vi "MGCC_FntStaMach_Error_State_handle.vi"() -> ()   [LabVIEW 2016]
uses:
  Error Handler Command Input.ctl
  Abnormal Fault State Control (He Yin)/Sub_VIs/Fault_Abnormal_state.vi
panel:
  in  "Boolean 2":bool
  out "Boolean":bool
  in  "Session in":refnum<k21>
  out "result":bool
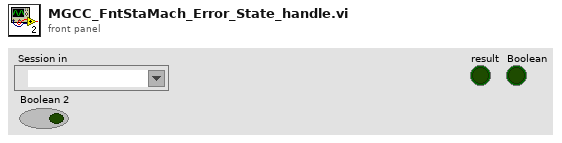
[diagram p1: front panel]
types:
  T1 = typedef "Error Handler Command Input.ctl" = enum16{"Initialize", "Handle Errors", "Report Errors"}
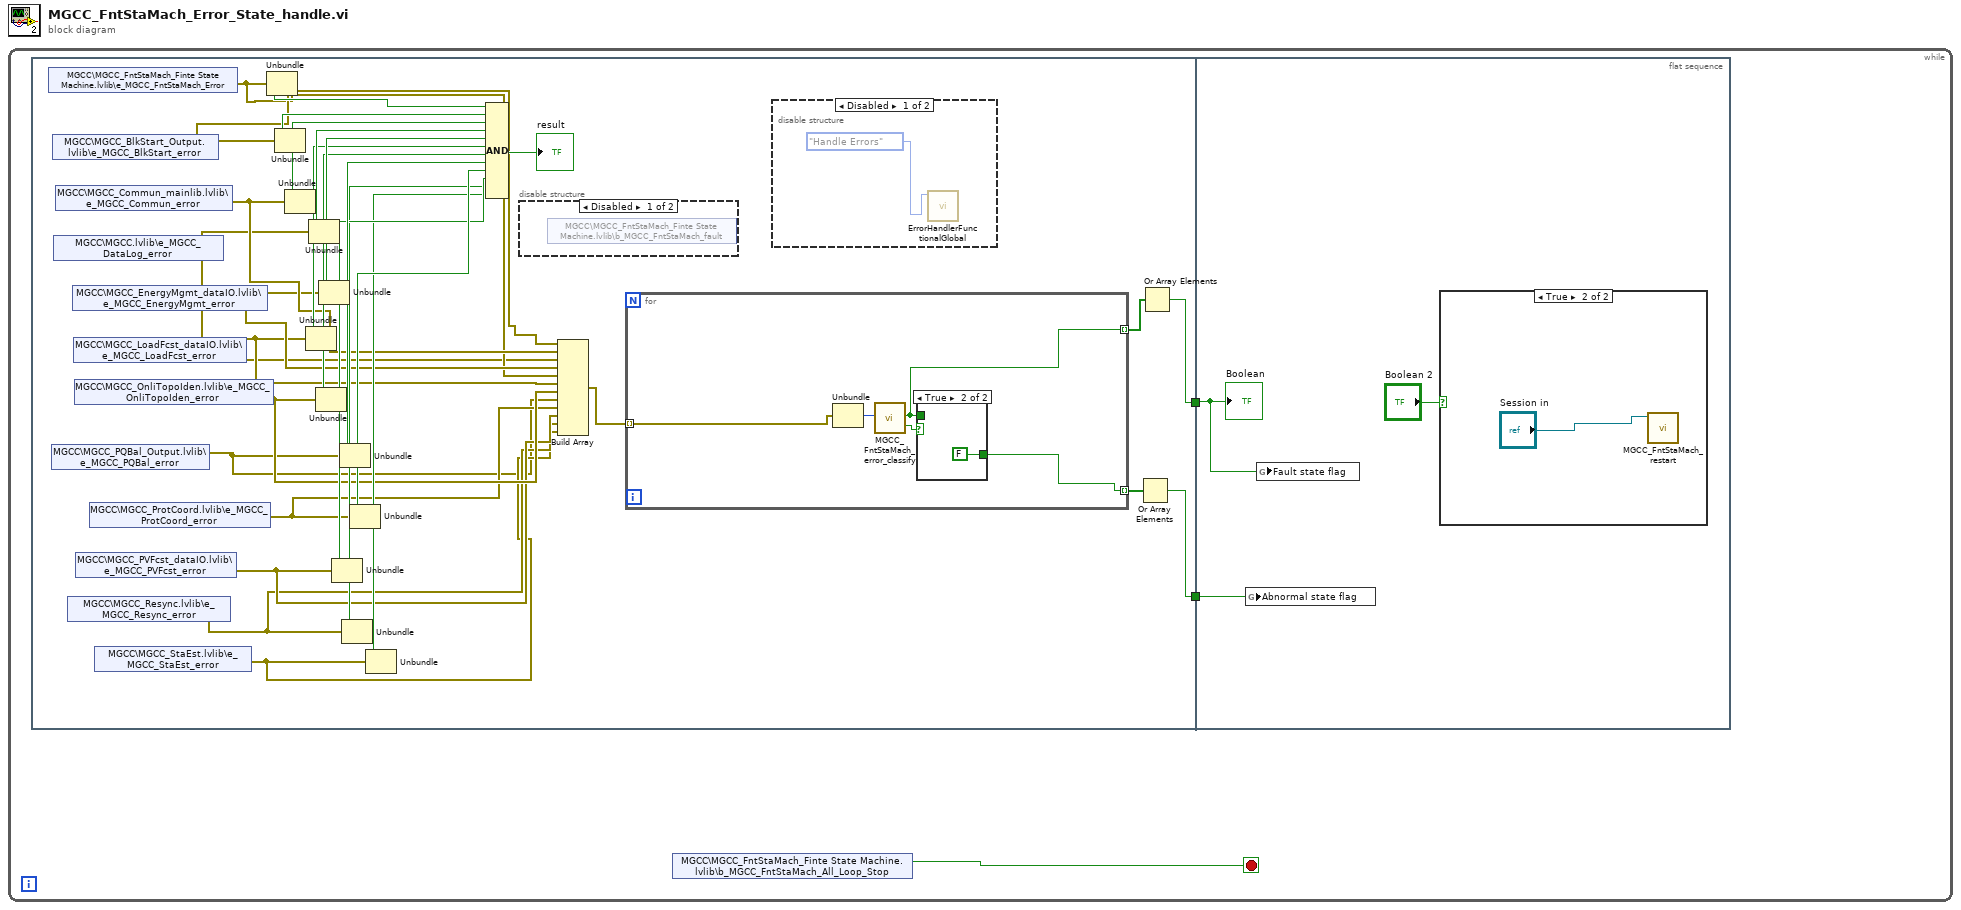
[diagram p0: block diagram]
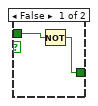
[diagram p3: hidden frame]
diagram:
  n1 = while {
    stop <- w3 stop-if-true
    n2 = flat-sequence {
      tunnel: [w5] -> w2
      tunnel: [w6] -> w1
      tunnel: w2 -> [w44]
      tunnel: w1 -> [w43]
      frame #0 {
        n3 = shared-variable "MGCC\\MGCC_FntStaMach_Finte State Machine.lvlib\\e_MGCC_FntStaMach_Error"() -> (w17:errorcluster)  [unwired: 1 in, 1 out]
        n4 = shared-variable "MGCC\\MGCC_PQBal_Output.lvlib\\e_MGCC_PQBal_error"() -> (w4:errorcluster)  [unwired: 1 in, 1 out]
        n5 = shared-variable "MGCC\\MGCC_BlkStart_Output.lvlib\\e_MGCC_BlkStart_error"() -> (w20:errorcluster)  [unwired: 1 in, 1 out]
        n6 = shared-variable "MGCC\\MGCC.lvlib\\e_MGCC_DataLog_error"() -> (w10:errorcluster)  [unwired: 1 in, 1 out]
        n7 = shared-variable "MGCC\\MGCC_Commun_mainlib.lvlib\\e_MGCC_Commun_error"() -> (w19:errorcluster)  [unwired: 1 in, 1 out]
        n8 = shared-variable "MGCC\\MGCC_Resync.lvlib\\e_MGCC_Resync_error"() -> (w12:errorcluster)  [unwired: 1 in, 1 out]
        n9 = shared-variable "MGCC\\MGCC_EnergyMgmt_dataIO.lvlib\\e_MGCC_EnergyMgmt_error"() -> (w18:errorcluster)  [unwired: 1 in, 1 out]
        n10 = shared-variable "MGCC\\MGCC_LoadFcst_dataIO.lvlib\\e_MGCC_LoadFcst_error"() -> (w16:errorcluster)  [unwired: 1 in, 1 out]
        n11 = shared-variable "MGCC\\MGCC_OnliTopoIden.lvlib\\e_MGCC_OnliTopoIden_error"() -> (w15:errorcluster)  [unwired: 1 in, 1 out]
        n12 = shared-variable "MGCC\\MGCC_PVFcst_dataIO.lvlib\\e_MGCC_PVFcst_error"() -> (w13:errorcluster)  [unwired: 1 in, 1 out]
        n13 = shared-variable "MGCC\\MGCC_ProtCoord.lvlib\\e_MGCC_ProtCoord_error"() -> (w14:errorcluster)  [unwired: 1 in, 1 out]
        n14 = shared-variable "MGCC\\MGCC_StaEst.lvlib\\e_MGCC_StaEst_error"() -> (w11:errorcluster)  [unwired: 1 in, 1 out]
        n15 = Unbundle(w17) -> ("status"=w33:bool)  [unwired: 2 out]
        n16 = Unbundle(w20) -> ("status"=w32:bool)  [unwired: 2 out]
        n17 = Unbundle(w19) -> ("status"=w31:bool)  [unwired: 2 out]
        n18 = Unbundle(w16) -> ("status"=w28:bool)  [unwired: 2 out]
        n19 = Unbundle(w10) -> ("status"=w30:bool)  [unwired: 2 out]
        n20 = Unbundle(w15) -> ("status"=w27:bool)  [unwired: 2 out]
        n21 = Unbundle(w18) -> ("status"=w29:bool)  [unwired: 2 out]
        n22 = Unbundle(w13) -> ("status"=w24:bool)  [unwired: 2 out]
        n23 = Unbundle(w4) -> ("status"=w26:bool)  [unwired: 2 out]
        n24 = Unbundle(w12) -> ("status"=w23:bool)  [unwired: 2 out]
        n25 = Unbundle(w14) -> ("status"=w25:bool)  [unwired: 2 out]
        n26 = Unbundle(w11) -> ("status"=w22:bool)  [unwired: 2 out]
        n27 = Compound Arithmetic op=AND(w33, w32, w31, w30, w29, w28, w27, w26, w25, w24, w23, w22) -> (→"result":bool)
        n28 = disable-structure shown="Disabled" {
          frame Disabled {
            n29 = shared-variable "MGCC\\MGCC_FntStaMach_Finte State Machine.lvlib\\b_MGCC_FntStaMach_fault"() -> ()  [unwired: 2 in, 1 out]
          }
          frame Enabled {
          }
        }
        n30 = Build Array(w20, w19, w10, w18, w17, w16, w15, w4, w14, w13, w12, w11) -> (w9:errorcluster[])
        n31 = for {
          tunnel: w9 -> [w37] mode=indexing
          tunnel: [w36] -> w8 mode=indexing
          tunnel: [w35] -> w7 mode=indexing
          n32 = Unbundle(w37) -> ("code"=w39:i32)  [unwired: 2 out]
          n33 = call "MGCC_FntStaMach_error_classify.vi"("Error"=w39) -> ("Error state"=w36:bool, "No error"=w38:bool)  [unwired: 17 in]
          n34 = case shown="True" w38 {
            tunnel: [w40 FALSE] -> w35
            tunnel: w36 -> [w41 _]
            frame False {
              n35 = Not(x=w41) -> (.not. x?=w40:bool)
            }
            frame True {
            }
          }
        }
        n36 = disable-structure shown="Disabled" {
          frame Disabled {
            n37 = call "ErrorHandlerFunctionalGlobal.vi"("Command Input"=Error_Handler_Command_Input."Handle Errors") -> ()  [unwired: 9 in, 2 out]
          }
          frame Enabled {
          }
        }
        n38 = Or Array Elements(Boolean array=w7) -> (logical OR=w6:bool)
        n39 = Or Array Elements(Boolean array=w8) -> (logical OR=w5:bool)
      }
      frame #1 {
        n40 = global write "Fault_Abnormal_state.vi" "Abnormal state flag"(w43) -> ()
        n41 = global write "Fault_Abnormal_state.vi" "Fault state flag"(w44) -> ()
        n42 = case shown="True" "Boolean 2" {
          frame False {
          }
          frame True {
            n43 = call "MGCC_FntStaMach_restart.vi"("Session in"="Session in") -> ()  [unwired: 8 in, 3 out]
          }
        }
        "Boolean" <- w44
      }
    }
    n44 = shared-variable "MGCC\\MGCC_FntStaMach_Finte State Machine.lvlib\\b_MGCC_FntStaMach_All_Loop_Stop"() -> (w3:bool)  [unwired: 1 in, 1 out]
  }
